vi "NI VeriStand - Remove Item Property.vi"(8 "error in (no error)":errorcluster, 10 "Property Name":string, 11 "Item Ref in":T1 format="%.0x") -> (0 "error out":errorcluster, 1 "Removed":bool, 3 "Item Ref out":T1 format="%.0x")   [LabVIEW 2026, in "Custom Devices Storage.lvlib"]
uses:
  Custom Devices Storage.lvlib
  <vilib>/NI VeriStand/Custom Device API/Custom Device Item Ref.ctl
  <vilib>/NI VeriStand/Custom Device API/Custom Device API.lvlib
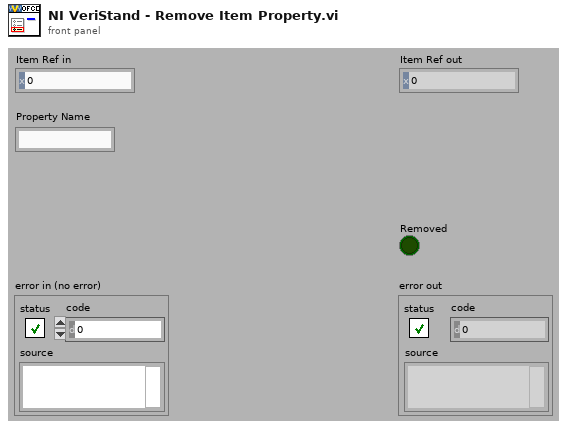
[diagram p1: front panel]
types:
  T1 = typedef "Custom Device API.lvlib/Custom Device Item Ref.ctl" = u64
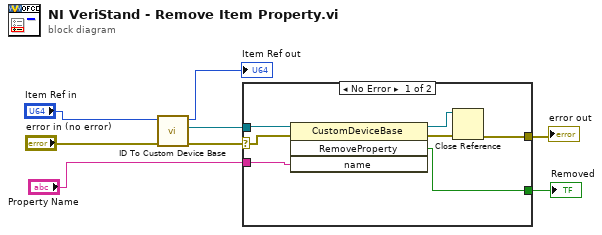
[diagram p0: block diagram]
diagram:
  n1 = call "ID To Custom Device Base.vi"("error in (no error)"="error in (no error)", "ID in"="Item Ref in") -> ("error out"=w5:errorcluster, "BaseNode"=w4:refnum<k39>, "ID out"=→"Item Ref out":u64)  [unwired: 7 in]
  n2 = case shown="No Error" w5 {
    selector: w5 -> [w14 w16]
    tunnel: w4 -> [w15 _]
    tunnel: "Property Name" -> [w11 _]
    tunnel: [w10 w16] -> w2
    tunnel: [w9 _] -> w1
    frame No Error {
      n3 = invoke class="CustomDeviceBase" method="RemoveProperty"(reference=w15, error in=w14, "name"=w11) -> (reference out=w12:refnum<k39>, error out=w13:errorcluster, "RemoveProperty"=w9:bool)  [unwired: 1 in, 1 out]
      n4 = Close Reference(reference=w12, error in (no error)=w13) -> (error out=w10:errorcluster)
    }
    frame Error {
    }
  }
  "error out" <- w2
  "Removed" <- w1
